vi "Read key-value pairs.vi"(8 "error in":errorcluster, 11 "NISE_CEF_serializable configuration in":refnum<class "NISE_CEF_serializable configuration.lvclass">) -> (0 "error out":errorcluster, 2 "key-value pairs":string[][](array[string]), 3 "NISE_CEF_serializable configuration out":refnum<class "NISE_CEF_serializable configuration.lvclass">)   [LabVIEW 2013, in "NISE_CEF_serializable configuration.lvclass"]
uses:
  NISE_CEF_serializable configuration.lvclass
  NISE_CEF_serializable configuration.lvclass/NISE_CEF_serializable configuration.ctl
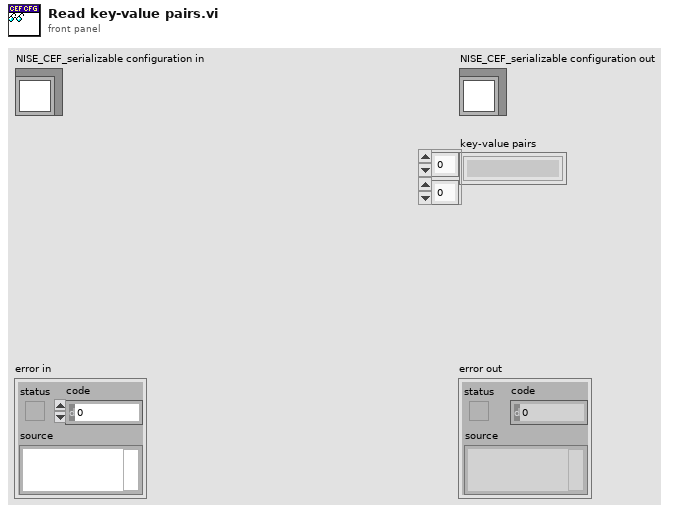
[diagram p1: front panel]
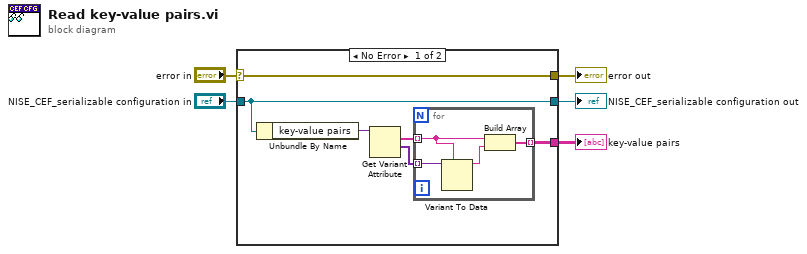
[diagram p0: block diagram]
diagram:
  n1 = case shown="No Error" "error in" {
    selector: "error in" -> [w11 w16]
    tunnel: [w11 w16] -> w4
    tunnel: [w10 w17] -> w2
    tunnel: "NISE_CEF_serializable configuration in" -> [w10 w17]
    tunnel: [w6 _] -> w1
    frame No Error {
      n2 = Unbundle By Name(w10) -> ("key-value pairs"=w9:variant)
      n3 = Get Variant Attribute(Variant=w9) -> (names=w8:string[], values=w7:variant[])  [unwired: 3 in, 2 out]
      n4 = for {
        tunnel: w8 -> [w15] mode=indexing
        tunnel: [w13] -> w6 mode=indexing
        tunnel: w7 -> [w12] mode=indexing
        n5 = Variant To Data(type=w15, Variant=w12) -> (data=w14:string)  [unwired: 1 in, 1 out]
        n6 = Build Array(w15, w14) -> (w13:string[])
      }
    }
    frame Error {
    }
  }
  "error out" <- w4
  "NISE_CEF_serializable configuration out" <- w2
  "key-value pairs" <- w1
